vi "Append Text Table to Report.vi"(0 "report in":refnum<class "NI_HTML.lvclass">, 1 "column width (1)":dbl=1.0 format="%.2f", 2 "measurement system":u16(ring)=2 caption="measurement system for column width (Default)" items=["US", "Metric", "Default"], 3 "MS Office parameters":T2, 5 "column headers":string[](array[string]), 7 "row headers":string[](array[string]), 9 "text data":string[][](array[string]), 11 "error in (no error)":errorcluster, 13 "separate page?":bool, 14 "show grid lines":bool=TRUE) -> (4 "report out":refnum<class "NI_HTML.lvclass">, 8 "range (wd) - start (xl)":T1, 10 "end (xl)":cluster{"row (xl) ":i32, "col (xl) ":i32}, 15 "error out":errorcluster)   [LabVIEW 2020, in "NI_HTML.lvclass"]
doc: "Appends a 2D array to a report as a table with the given column width. You can use this polymorphic VI to append an array of strings or numbers. The data type you wire to the <B>text data</B> input determines the polymorphic instance to use."
uses:
  <vilib>/Utility/NIReport.llb/HTML/NI_HTML.lvclass
  <vilib>/Utility/NIReport.llb/HTML/NI_HTML.lvclass/NI_HTML.ctl
  <vilib>/Utility/NIReport.llb/NI_ReportGenerationCore.lvlib
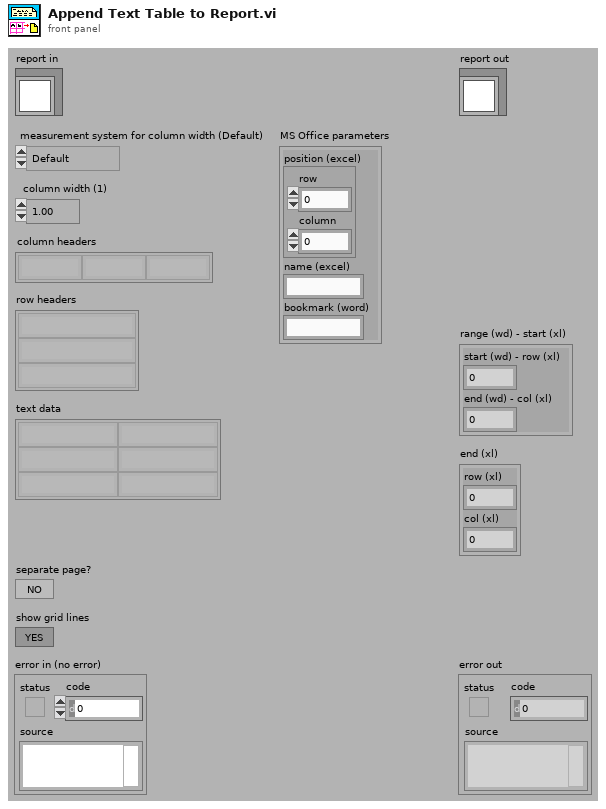
[diagram p1: front panel]
types:
  T1 = cluster{"start (wd) - row (xl) ":i32, "end (wd) - col (xl) ":i32}
  T2 = cluster{"position (excel)":cluster{"row":i32, "column":i32}, "name (excel)":string, "bookmark (word)":string}
  T3 = typedef "NI_ReportGenerationCore.lvlib/HTML Report Data.ctl" = cluster{"Body Text":string, "Font Tag":string, "Title Text":string, "Header Text":string, "Footer Text":string, "Image List":path[]}
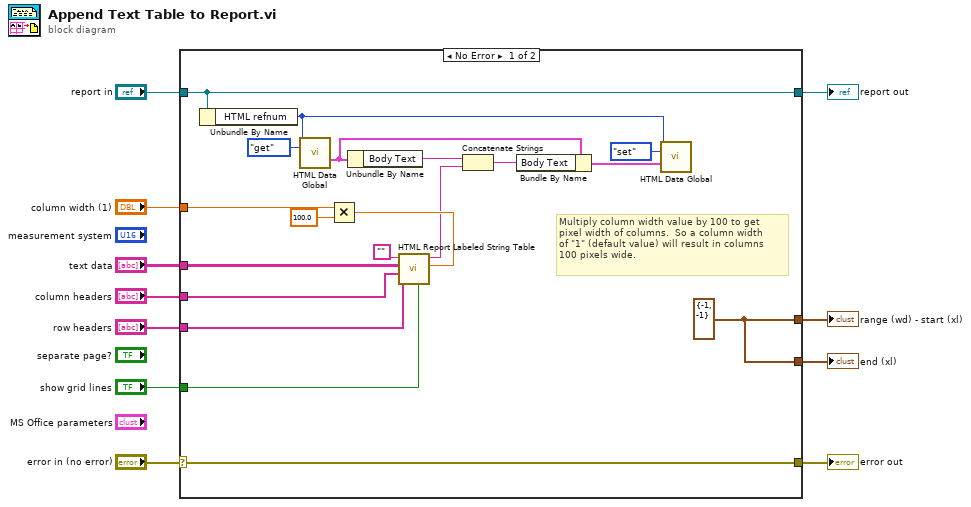
[diagram p0: block diagram]
diagram:
  n1 = case shown="No Error" "error in (no error)" {
    selector: "error in (no error)" -> [w30 w32]
    tunnel: [w30 w32] -> w10
    tunnel: [w17 w31] -> w8
    tunnel: "report in" -> [w17 w31]
    tunnel: [w24 _] -> w7
    tunnel: [w24 _] -> w6
    tunnel: "show grid lines" -> [w23 _]
    tunnel: "text data" -> [w22 _]
    tunnel: "column headers" -> [w21 _]
    tunnel: "row headers" -> [w20 _]
    tunnel: "column width (1)" -> [w19 _]
    frame No Error {
      w24 = cluster{"row (xl)":i32, "col (xl)":i32} {"row (xl)"=-1, "col (xl)"=-1} ("end (xl)")
      # "Multiply column width value by 100 to get\npixel width of columns.  So a column width\nof \"1\" (default value) will result in columns\n100 pixels wide."
      n2 = Unbundle By Name(w17) -> ("HTML refnum"=w12:u32)
      n3 = call <vilib>:"HTML Data Global.vi"("HTML refnum"=w12, "menu"=enum16{"init", "get", "set", "delete"}."get") -> ("HTML report data out"=w13:T3)  [unwired: 1 in, 12 out]
      n4 = Multiply(x=w19, y=100.0) -> (x*y=w29:dbl)
      n5 = Unbundle By Name(w13) -> ("Body Text"=w25:string)
      n6 = call <vilib>:"HTML Report Labeled String Table.vi"("column width (100)"=w29, "Show Grid"=w23, "row headers"=w20, "column headers"=w21, "table contents"=w22, "HTML in"="") -> ("HTML out"=w26:string)  [unwired: 2 in, 3 out]
      n7 = Concatenate Strings(w25, w26) -> (w14:string)
      n8 = Bundle By Name(cluster=w13, "Body Text"=w14) -> (w15:T3)
      n9 = call <vilib>:"HTML Data Global.vi"("HTML refnum"=w12, "menu"=enum16{"init", "get", "set", "delete"}."set", "HTML report data in"=w15) -> ()  [unwired: 13 out]
    }
    frame Error {
    }
  }
  "error out" <- w10
  "report out" <- w8
  "end (xl)" <- w6
  "range (wd) - start (xl)" <- w7
